vi "test_Set-Get Protocol Error.vi"(8 "error in (no error)":errorcluster, 11 "TestCase in":refnum<class "Instrument Addon Scripting API Custom Device Unit Tests.lvclass">) -> (0 "error out":errorcluster, 3 "TestCase out":refnum<class "Instrument Addon Scripting API Custom Device Unit Tests.lvclass">)   [LabVIEW 2019, in "Instrument Addon Scripting API Custom Device Unit Tests.lvclass"]
uses:
  Instrument Addon Scripting API Custom Device Unit Tests.lvclass
  Includes/Protocols.lvlibp/Protocol Parent/Protocol Parent.lvclass
  Instrument Addon Scripting API Custom Device Unit Tests.lvclass/Instrument Addon Scripting API Custom Device Unit Tests.ctl
  <vilib>/addons/_JKI Toolkits/VI Tester/TestCase.llb/TestCase.lvclass
  APIs/Scripting API/Instrument Addon Scripting API.lvlib
  C:/Program Files (x86)/National Instruments/LabVIEW 2019/vi.lib/addons/_JKI Toolkits/VI Tester/TestCase.llb/TestCase.lvclass
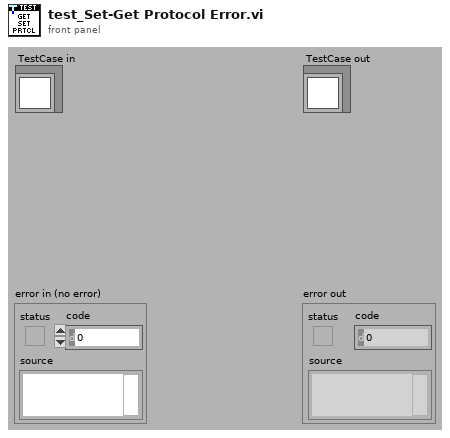
[diagram p1: front panel]
types:
  T1 = typedef "Custom Device API.lvlib/Custom Device Item Ref.ctl" = u64
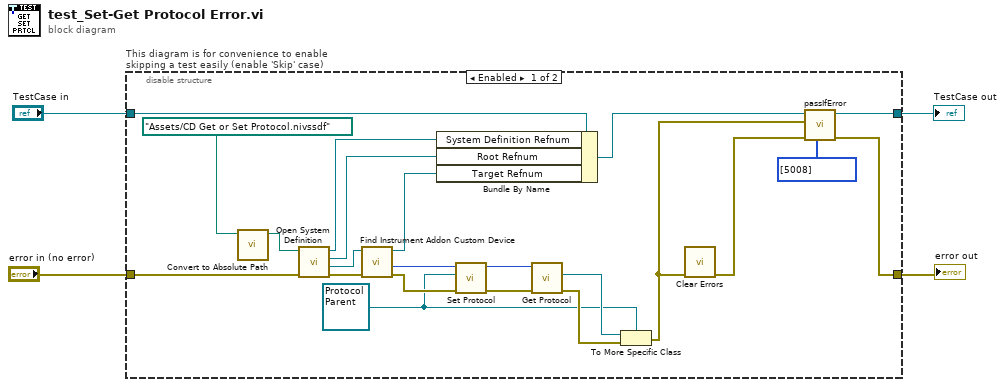
[diagram p0: block diagram]
diagram:
  n1 = disable-structure "This diagram is for convenience to enable skipping a test easily (enable 'Skip' case)" shown="Enabled" {
    disable-tunnel: "TestCase in" -> [w9 w30]
    disable-tunnel: [w13 w28] -> w1
    disable-tunnel: [w10 w29] -> w3
    disable-tunnel: "error in (no error)" -> [w26 w27]
    frame Enabled {
      w14 = refnum<class "Protocol Parent.lvclass"> refnum ("Protocols.lvlibp:Protocol Parent.lvclass")
      n2 = call "Convert to Absolute Path.vi"("System Definition File"=path "Assets/CD Get or Set Protocol.nivssdf" ("SDF file")) -> ("Absolute Path"=w24:path)  [unwired: 10 in]
      n3 = call "Open System Definition.vi"("error in (no error)"=w26, "System Definition File"=w24) -> ("error out"=w23:errorcluster, "Target Refnum"=w22:refnum<k24>, "Root Refnum"=w6:refnum<k24>, "System Definition Refnum"=w7:refnum<k24>)  [unwired: 6 in]
      n4 = call "Find Instrument Addon Custom Device.vi"("error in"=w23, "target in"=w22) -> ("error out"=w21:errorcluster, "NodeID"=w20:u64, "target out"=w5:refnum<k24>)  [unwired: 7 in]
      n5 = Bundle By Name(cluster=w9, "System Definition Refnum"=w7, "Root Refnum"=w6, "Target Refnum"=w5) -> (w8:refnum<class "Instrument Addon Scripting API Custom Device Unit Tests.lvclass">)
      n6 = call "Set Protocol.vi"("error in (no error)"=w21, "protocol"=w14, "instrument addon refnum in"=w20) -> ("error out"=w18:errorcluster, "instrument addon refnum out"=w19:T1)  [unwired: 7 in]
      n7 = call "Get Protocol.vi"("error in (no error)"=w18, "instrument addon refnum in"=w19) -> ("error out"=w16:errorcluster, "protocol"=w17:refnum<class "Protocol Parent.lvclass">)  [unwired: 7 in, 1 out]
      n8 = To More Specific Class(target class=w14, reference=w17, error in=w16) -> (error out=w15:errorcluster)  [unwired: 1 out]
      n9 = call <vilib>:"Clear Errors.vi"("error in (no error)"=w15) -> ("error out"=w11:errorcluster)  [unwired: 5 in, 1 out]
      n10 = call-dynamic "passIfError.vi"("passing error codes (default = any error code)"=i32[] [5008], "error in (no error)"=w11, "error"=w15, "TestCase in"=w8) -> ("error out"=w10:errorcluster, "TestCase out"=w13:refnum<class "Instrument Addon Scripting API Custom Device Unit Tests.lvclass">)  [unwired: 6 in]
    }
    frame Disabled {
      # "skip test result while test is under development"
      n11 = call <vilib>:"skip.vi"("error in (no error)"=w27, "TestCase in"=w30) -> ("error out"=w29:errorcluster, "TestCase out"=w28:refnum<class "Instrument Addon Scripting API Custom Device Unit Tests.lvclass">)  [unwired: 8 in]
    }
  }
  "error out" <- w3
  "TestCase out" <- w1
